vi "Get INI file Path.vi"(4 "error in (no error)":errorcluster) -> (0 "error out":errorcluster, 3 "appended path":path)   [LabVIEW 2015, in "Config Data.lvlib" / "Config Data.lvclass"]
uses:
  Config Data.lvclass
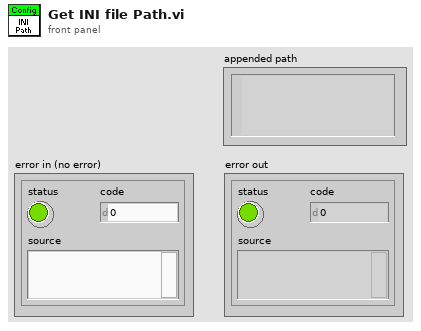
[diagram p1: front panel]
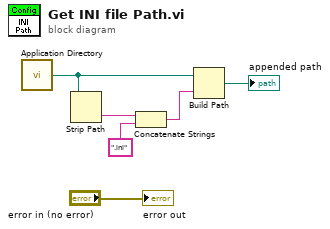
[diagram p0: block diagram]
diagram:
  n1 = call <vilib>:"Application Directory.vi"() -> ("Application Directory"=w2:path)
  n2 = Strip Path(path=w2) -> (name=w1:string)  [unwired: 1 out]
  n3 = Concatenate Strings(w1, ".ini") -> (w5:string)
  n4 = Build Path(base path=w2, name or relative path=w5) -> (appended path=→"appended path":path)
  "error out" <- "error in (no error)"
